vi "Final_DAQ_v1.vi"() -> ()   [LabVIEW 2019]
uses:
  src/class/mqtt/mqttTXqueue/mqttTXdataQueueFunction.ctl
  src/class/mqtt/mqttTXqueue/mqttRXsubscriptionEventFunction.ctl
  src/class/mqtt/mqtt.lvclass
panel:
  out "電暖爐":bool
  out "電扇":bool
  out "電燈":bool
  out "開門 Flag":bool
  out "電暖爐-M":bool
  out "電扇-M":bool
  out "開門":bool
  out "電燈-M":bool
  out "溫度過低":bool
  out "溫度過高":bool
  out "Boolean":bool
  out "old-temp":dbl
  out "Numeric 2":dbl
  out "subscripts-status":bool
  out "Publish Topic":string
  out "Publish Data":string
  out "溫度上限(*C)":dbl
  out "溫度下限(*C)":dbl
  out "Subscripts Topic":string
  out "Subscripts Data":string
  out "F-format string":string
  out "now-temp":dbl
  out "Thermometer":dbl(slide) scale=0.0..40.0
  in  "stop":bool
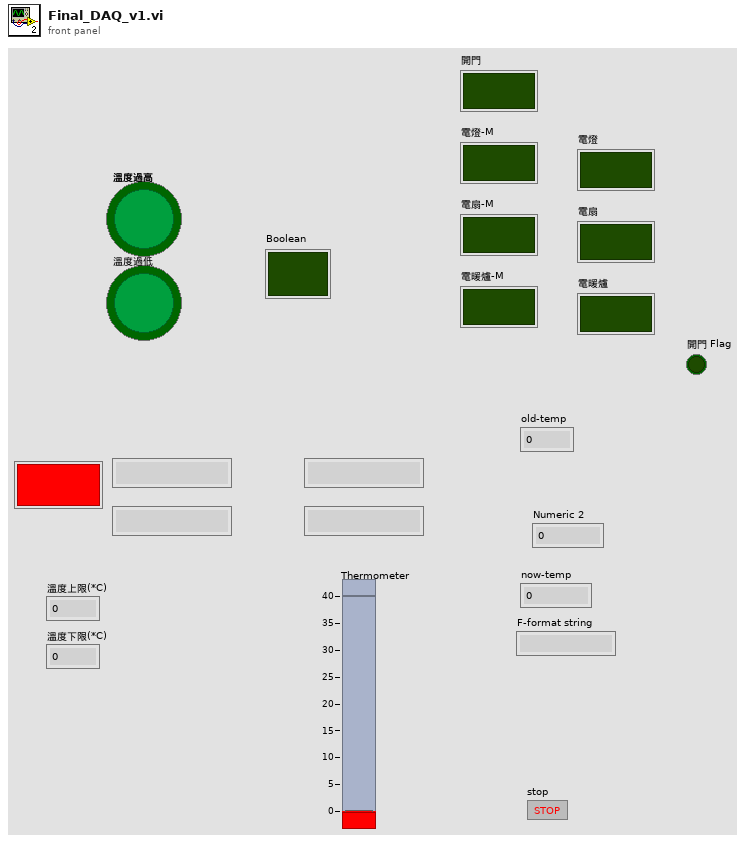
[diagram p1: front panel]
types:
  T1 = typedef "mqttRXsubscriptionEventFunction.ctl" = enum16{"init", "deinit", "getEventRef", "event"}
  T2 = typedef "mqttTXdataQueueFunction.ctl" = enum16{"init", "deinit", "getQueue", "enqueue"}
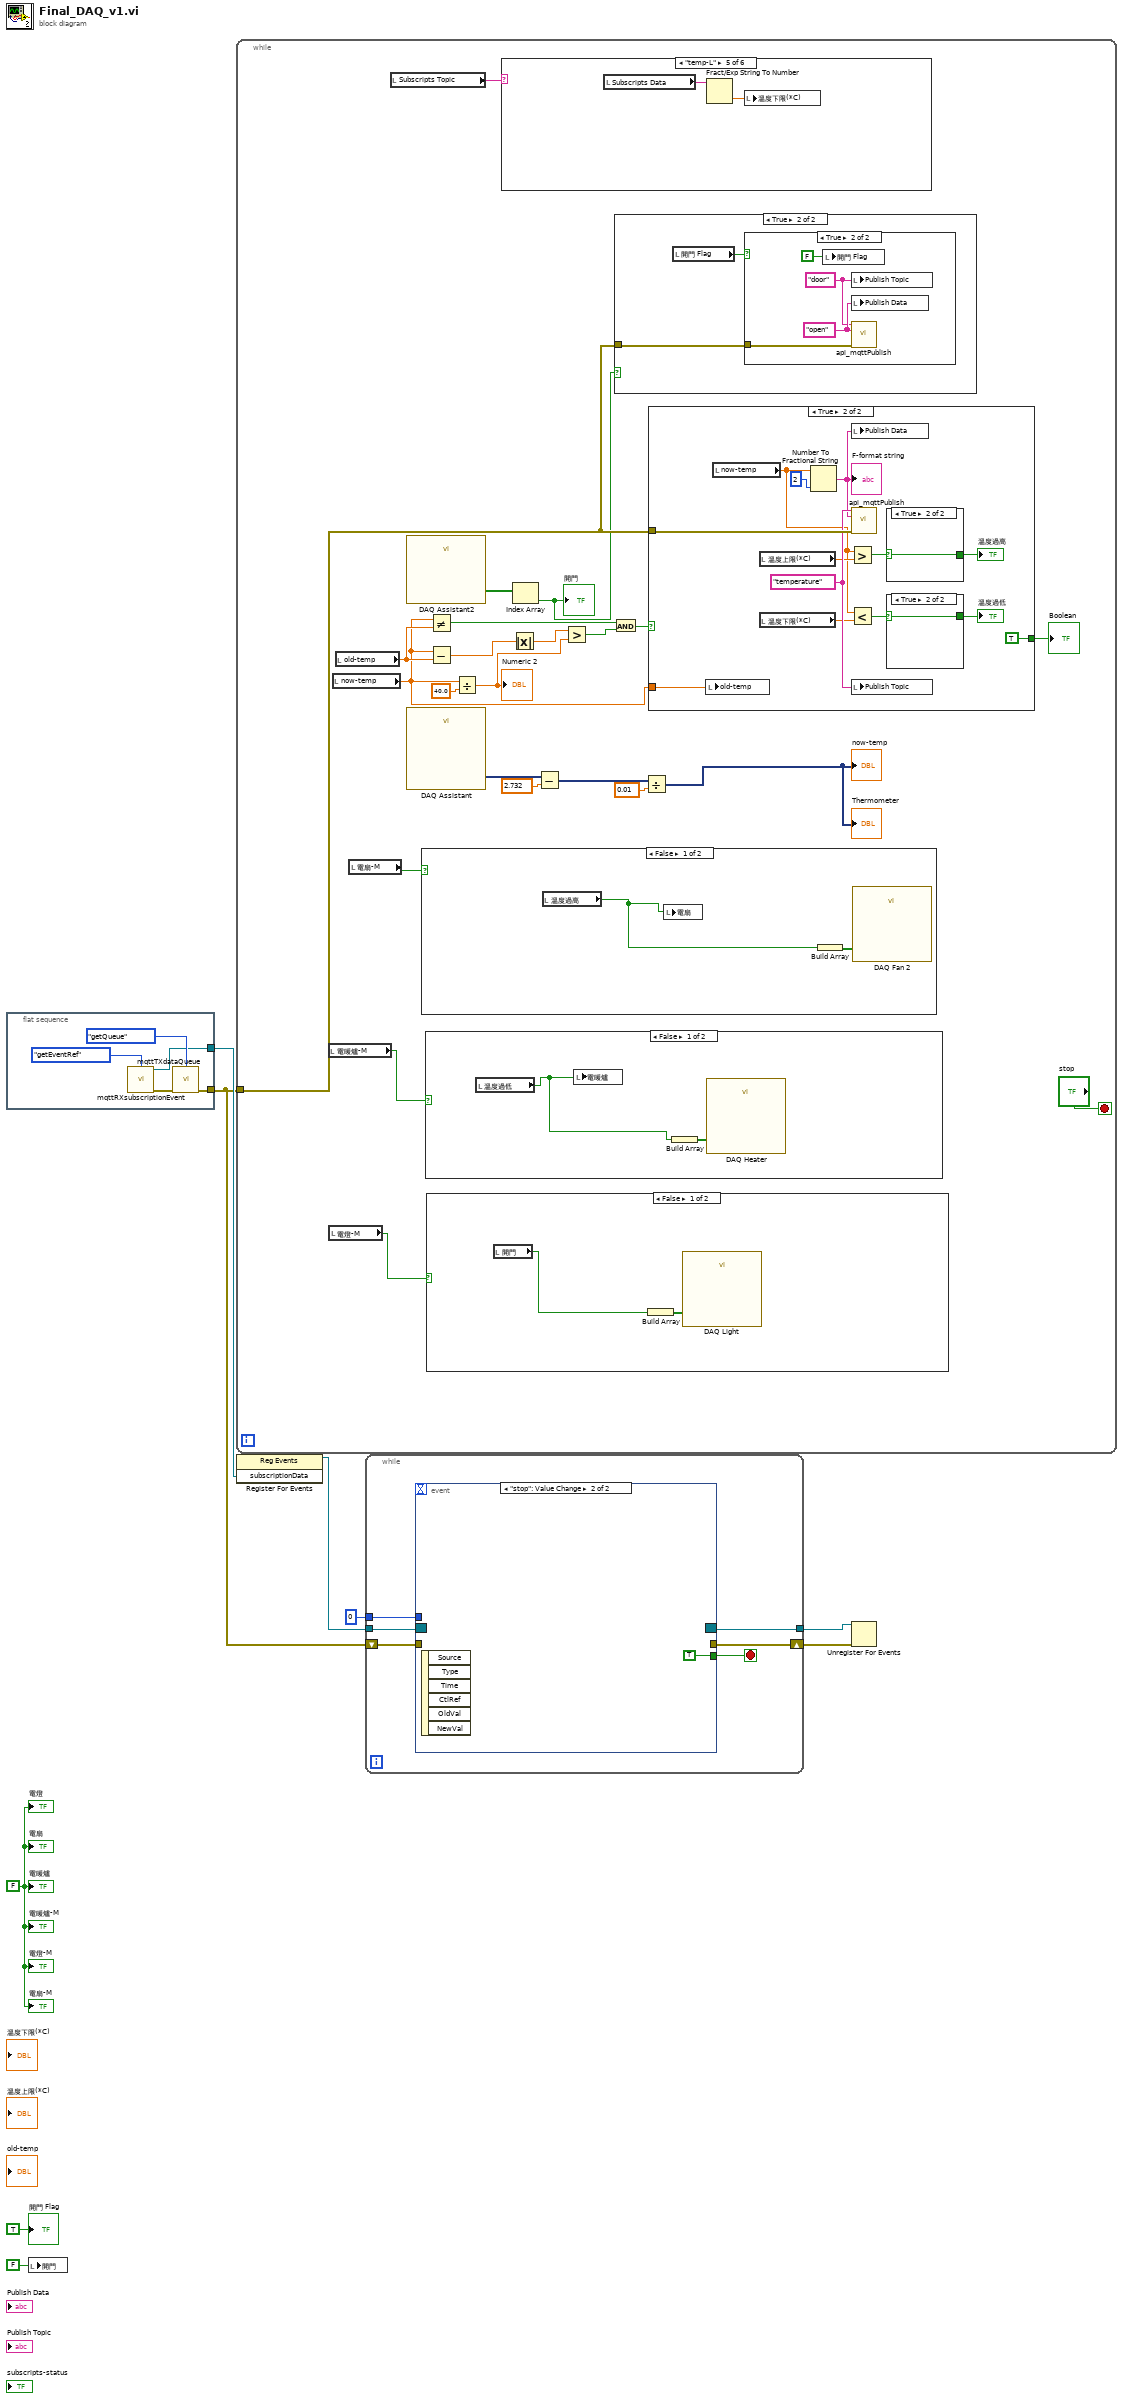
[diagram p0: block diagram]
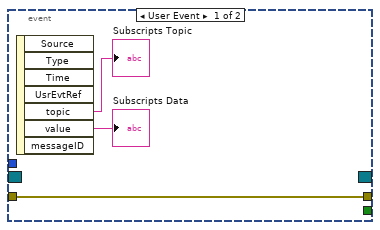
[diagram p2: hidden frame]
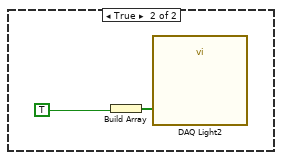
[diagram p3: hidden frame]
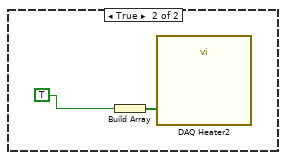
[diagram p4: hidden frame]
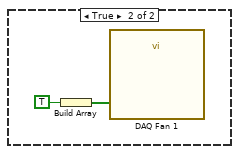
[diagram p5: hidden frame]
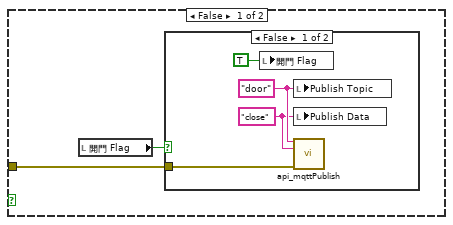
[diagram p6: hidden frame]
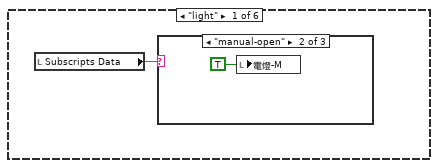
[diagram p9: hidden frame]
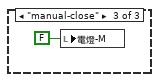
[diagram p11: hidden frame]
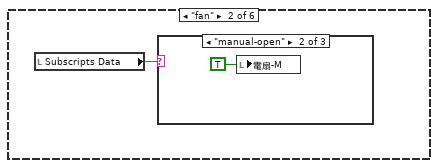
[diagram p12: hidden frame]
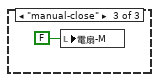
[diagram p14: hidden frame]
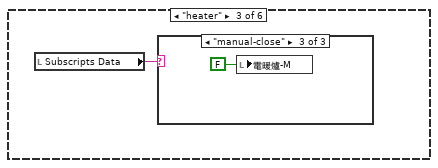
[diagram p15: hidden frame]
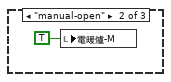
[diagram p17: hidden frame]
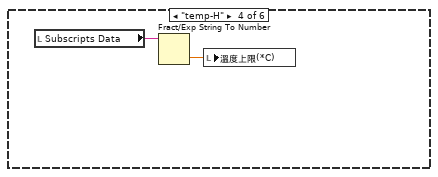
[diagram p18: hidden frame]
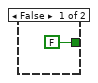
[diagram p20: hidden frame]
diagram:
  w1 = FALSE
  n1 = flat-sequence {
    tunnel: [w13] -> w4
    tunnel: [w10] -> w9
    frame #0 {
      n2 = call "mqttRXsubscriptionEvent.vi"("function"=mqttRXsubscriptionEventFunction."getEventRef") -> ("subscriptionData"=w10:refnum<user-event>, "error out"=w12:errorcluster)  [unwired: 13 in]
      n3 = call "mqttTXdataQueue.vi"("function"=mqttTXdataQueueFunction."getQueue", "error in (no error)"=w12) -> ("error out"=w13:errorcluster)  [unwired: 12 in, 1 out]
    }
  }
  n4 = local write "開門"(FALSE ("開門")) -> ()
  n5 = while {
    tunnel: w4 -> [w20]
    stop <- "stop" stop-if-true
    n6 = local read "電暖爐-M"() -> (w17:bool)
    n7 = local read "電燈-M"() -> (w16:bool)
    n8 = local read "now-temp"() -> (w24:dbl)
    n9 = local read "old-temp"() -> (w30:dbl)
    n10 = local read "電扇-M"() -> (w18:bool)
    n11 = local read "Subscripts Topic"() -> (w21:string)
    n12 = call "DAQ Assistant2"() -> ("data"=w32:bool[])  [unwired: 17 in, 2 out]
    n13 = call "DAQ Assistant"() -> ("data"=w33:dynamicdata)  [unwired: 17 in, 2 out]
    n14 = case shown="False" w18 {
      frame False {
        n15 = local read "溫度過高"() -> (w46:bool)
        n16 = local write "電扇"(w46) -> ()
        n17 = Build Array(w46) -> (w47:bool[])
        n18 = call "DAQ Fan 2"("data"=w47) -> ()  [unwired: 17 in, 2 out]
      }
      frame True {
        n19 = Build Array(TRUE) -> (w49:bool[])
        n20 = call "DAQ Fan 1"("data"=w49) -> ()  [unwired: 17 in, 2 out]
      }
    }
    n21 = case shown="False" w17 {
      frame False {
        n22 = local read "溫度過低"() -> (w43:bool)
        n23 = local write "電暖爐"(w43) -> ()
        n24 = Build Array(w43) -> (w42:bool[])
        n25 = call "DAQ Heater"("data"=w42) -> ()  [unwired: 17 in, 2 out]
      }
      frame True {
        n26 = Build Array(TRUE) -> (w44:bool[])
        n27 = call "DAQ Heater2"("data"=w44) -> ()  [unwired: 17 in, 2 out]
      }
    }
    n28 = case shown="False" w16 {
      frame False {
        n29 = local read "開門"() -> (w39:bool)
        n30 = Build Array(w39) -> (w38:bool[])
        n31 = call "DAQ Light"("data"=w38) -> ()  [unwired: 17 in, 2 out]
      }
      frame True {
        n32 = Build Array(TRUE) -> (w40:bool[])
        n33 = call "DAQ Light2"("data"=w40) -> ()  [unwired: 17 in, 2 out]
      }
    }
    n34 = Not Equal?(x=w24, y=w30) -> (x != y?=w31:bool)
    n35 = Subtract(x=w24, y=w30) -> (x-y=w29:dbl)
    n36 = Divide(x=w24, y=40.0) -> (x/y=w27:dbl)
    "Numeric 2" <- w27
    n37 = case shown="\"temp-L\"" w21 {
      frame "light" {
        n38 = local read "Subscripts Data"() -> (w62:string)
        n39 = case shown="\"manual-open\"" w62 {
          frame "None", Default {
          }
          frame "manual-open" {
            n40 = local write "電燈-M"(TRUE ("電燈")) -> ()
          }
          frame "manual-close" {
            n41 = local write "電燈-M"(FALSE ("電燈")) -> ()
          }
        }
      }
      frame "fan" {
        n42 = local read "Subscripts Data"() -> (w65:string)
        n43 = case shown="\"manual-open\"" w65 {
          frame "None", Default {
          }
          frame "manual-open" {
            n44 = local write "電扇-M"(TRUE ("電扇")) -> ()
          }
          frame "manual-close" {
            n45 = local write "電扇-M"(FALSE ("電扇")) -> ()
          }
        }
      }
      frame "heater" {
        n46 = local read "Subscripts Data"() -> (w68:string)
        n47 = case shown="\"manual-close\"" w68 {
          frame "None", Default {
          }
          frame "manual-open" {
            n48 = local write "電暖爐-M"(TRUE ("電暖爐")) -> ()
          }
          frame "manual-close" {
            n49 = local write "電暖爐-M"(FALSE ("電暖爐")) -> ()
          }
        }
      }
      frame "temp-H" {
        n50 = local read "Subscripts Data"() -> (w72:string)
        n51 = Fract/Exp String To Number(string=w72) -> (number=w71:dbl)  [unwired: 3 in, 1 out]
        n52 = local write "溫度上限(*C)"(w71) -> ()
      }
      frame "temp-L" {
        n53 = local read "Subscripts Data"() -> (w74:string)
        n54 = Fract/Exp String To Number(string=w74) -> (number=w73:dbl)  [unwired: 3 in, 1 out]
        n55 = local write "溫度下限(*C)"(w73) -> ()
      }
      frame "none", Default {
      }
    }
    n56 = Absolute Value(x=w29) -> (abs(x)=w28:dbl)
    n57 = Index Array(array=w32) -> (element=w19:bool)  [unwired: 1 in]
    "開門" <- w19
    n58 = Subtract(x=w33, y=2.732) -> (x-y=w35:dynamicdata)
    n59 = Greater?(x=w28, y=w27) -> (0:w26:bool)
    n60 = And(x=w31, y=w26) -> (x .and. y?=w25:bool)
    n61 = case shown="True" w19 {
      tunnel: w20 -> [w50 w57]
      frame False {
        n62 = local read "開門 Flag"() -> (w51:bool)
        n63 = case shown="False" w51 {
          tunnel: w50 -> [w52 _]
          frame False {
            w53 = "close"
            w54 = "door"
            n64 = local write "開門 Flag"(TRUE ("開門 Flag")) -> ()
            n65 = local write "Publish Topic"(w54) -> ()
            n66 = local write "Publish Data"(w53) -> ()
            n67 = call "api_mqttPublish.vi"("topic"=w54, "value"=w53, "error in (no error)"=w52) -> ()  [unwired: 11 in, 2 out]
          }
          frame True {
          }
        }
      }
      frame True {
        n68 = local read "開門 Flag"() -> (w56:bool)
        n69 = case shown="True" w56 {
          tunnel: w57 -> [_ w59]
          frame False {
          }
          frame True {
            w61 = "open" ("value")
            w60 = "door" ("topic")
            n70 = local write "開門 Flag"(FALSE ("開門 Flag")) -> ()
            n71 = local write "Publish Topic"(w60) -> ()
            n72 = local write "Publish Data"(w61) -> ()
            n73 = call "api_mqttPublish.vi"("topic"=w60, "value"=w61, "error in (no error)"=w59) -> ()  [unwired: 11 in, 2 out]
          }
        }
      }
    }
    n74 = Divide(x=w35, y=0.01) -> (x/y=→"Thermometer" →"now-temp":dynamicdata)
    n75 = case shown="True" w25 {
      tunnel: w24 -> [_ w88]
      tunnel: [FALSE ("Boolean") TRUE ("Boolean")] -> w23
      tunnel: w20 -> [_ w86]
      frame False {
      }
      frame True {
        w84 = "temperature" ("topic")
        n76 = local write "old-temp"(w88) -> ()
        n77 = local read "now-temp"() -> (w78:dbl)
        n78 = local read "溫度上限(*C)"() -> (w82:dbl)
        n79 = local read "溫度下限(*C)"() -> (w79:dbl)
        n80 = Number To Fractional String(number=w78, precision (6)=i16 2) -> (F-format string=w83:string)  [unwired: 2 in]
        "F-format string" <- w83
        n81 = Greater?(x=w78, y=w82) -> (0:w81:bool)
        n82 = Less?(x=w78, y=w79) -> (x < y?=w80:bool)
        n83 = local write "Publish Data"(w83) -> ()
        n84 = call "api_mqttPublish.vi"("topic"=w84, "value"=w83, "error in (no error)"=w86) -> ()  [unwired: 11 in, 2 out]
        n85 = local write "Publish Topic"(w84) -> ()
        n86 = case shown="True" w81 {
          selector: w81 -> [w91 w92]
          tunnel: [w91 w92] -> w77
          frame False {
          }
          frame True {
          }
        }
        "溫度過高" <- w77
        n87 = case shown="True" w80 {
          selector: w80 -> [w89 w90]
          tunnel: [w89 w90] -> w76
          frame False {
          }
          frame True {
          }
        }
        "溫度過低" <- w76
      }
    }
    "Boolean" <- w23
  }
  n88 = register-events(w9) -> (reference out=w8:refnum<event-registration>)  [unwired: 2 in, 1 out]
  n89 = while {
    tunnel: w8 -> [w95]
    shift-right: [w96] -> w7
    shift-left: w4 -> [w97]
    tunnel: [w94] -> w6
    tunnel: 0 -> [w93]
    stop <- w98 stop-if-true
    n90 = event shown="[1] \"stop\": Value Change" {
      selector: w95 -> [_ _]
      dyn-events: [_ _] -> w94
      timeout: _ -> [_ _]
      tunnel: [_ TRUE] -> w98
      tunnel: w97 -> [w99 _]
      tunnel: [w99 _] -> w96
      tunnel: w93 -> [_ _]
      event User Event {
        n91 = event-data() -> ("topic"=→"Subscripts Topic":string, "value"=→"Subscripts Data":string)  [unwired: 1 in, 5 out]
      }
      event "stop": Value Change {
        n92 = event-data() -> ()  [unwired: 1 in, 6 out]
      }
    }
  }
  n93 = Unregister For Events(event registration refnum=w6, error in=w7) -> ()  [unwired: 1 out]
  "電扇-M" <- w1
  "電暖爐-M" <- w1
  "電燈-M" <- w1
  "開門 Flag" <- TRUE ("開門 Flag")
  "電燈" <- w1
  "電扇" <- w1
  "電暖爐" <- w1
